vi "Instrument Manager Loop.vi"(8 "System Control":refnum<queue>, 11 "Optimizer Manager":refnum<queue>) -> (0 "error out":errorcluster)   [LabVIEW 2020, in "SQSnobFit Control Panel.lvlib" / "Instrument Manager.lvlib"]
uses:
  Instrument Manager/Instrument Manager.lvlib
  support/Message Queue/Message Cluster.ctl
  Instrument Manager/Instrument State.ctl
  <vilib>/addons/zeromq/zmq_context.lvclass
  <vilib>/addons/zeromq/zmq_socket.lvclass
  <vilib>/addons/zeromq/socket_type.ctl
  <vilib>/addons/zeromq/poll_type.ctl
  Typedefs/Best Result.ctl
  <vilib>/Utility/error.llb/Error Cluster From Error Code.vi
  <vilib>/addons/zeromq/zmq_poll_scalar.vi
  <vilib>/ErrorRing/Error Ring.xnode
  support/Message Queue/Message Queue.lvlib
  SQSnobFit Control Panel.lvlib
  <vilib>/addons/zeromq/zeromq.lvlib
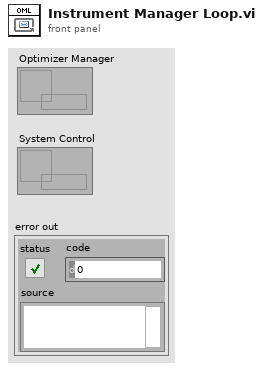
[diagram p1: front panel]
types:
  T1 = typedef "zeromq.lvlib/socket_type.ctl" = enum8{"ZMQ_PAIR", "ZMQ_PUB", "ZMQ_SUB", "ZMQ_REQ", "ZMQ_REP", "ZMQ_DEALER", "ZMQ_ROUTER", "ZMQ_PULL", "ZMQ_PUSH", "ZMQ_XPUB", "ZMQ_XSUB"}
  T2 = typedef "SQSnobFit Control Panel.lvlib/Instrument Manager.lvlib/Instrument State.ctl" = cluster{"Context":refnum<class "zmq_context.lvclass">, "Socket":refnum<class "zmq_socket.lvclass">, "Running Since":timestamp, "New Parameters (values)":cluster{"Time Stamp":timestamp, "Name":string[], "Value":dbl[]}, "Optimizer Path":path, "Running":bool, "Response Counter":u8, "Response Timeout (ms)":u32, "Response Retries":u32, "Endpoint":string, "Starting up?":bool, "New Parameters (percents)":cluster{"Time Stamp":timestamp, "Name":string[], "Value":dbl[]}, "Flow Rate Constant":dbl, "Yield":dbl, "Current Best (values)":cluster{"Parameter Names":string[], "Parameter Values":dbl[], "Function Value":dbl}}
  T3 = typedef "zeromq.lvlib/poll_type.ctl" = enum16{"None", "In", "Out", "In/Out"}
  T4 = typedef "SQSnobFit Control Panel.lvlib/Best Result.ctl" = cluster{"value":dbl, "parameters":dbl[], "history":dbl[][], "steps":dbl}
  T5 = cluster{"seconds since 1Jan1904":timestamp, string[], dbl[]}
  T6 = cluster{"Time Stamp":timestamp, "Name":string[], "Value":dbl[]}
  T7 = typedef "zeromq.lvlib/error_type.ctl" = enum16{"No Error", "EUNKNOWN", "ENOTSUP", "EPROTONOSUPPORT", "ENOBUFS", "ENETDOWN", "EADDRINUSE", "EADDRNOTAVAIL", "ECONNREFUSED", "EINPROGRESS", "ENOTSOCK", "EMSGSIZE", "EAFNOSUPPORT", "ENETUNREACH", "ECONNABORT", "ECONNRESET", "ENOTCONN", "ETIMEDOUT", "EHOSTUNREACH", "ENETRESET", "EBUSY", "EINVAL", "ENODEV", "EFAULT", "EINTR", "ENOENT", "ENOMEM", "EAGAIN", "EMFILE", "EFSM", "ENOCOMPATPROTO", "ETERM", "EMTHREAD", "Invalid"}
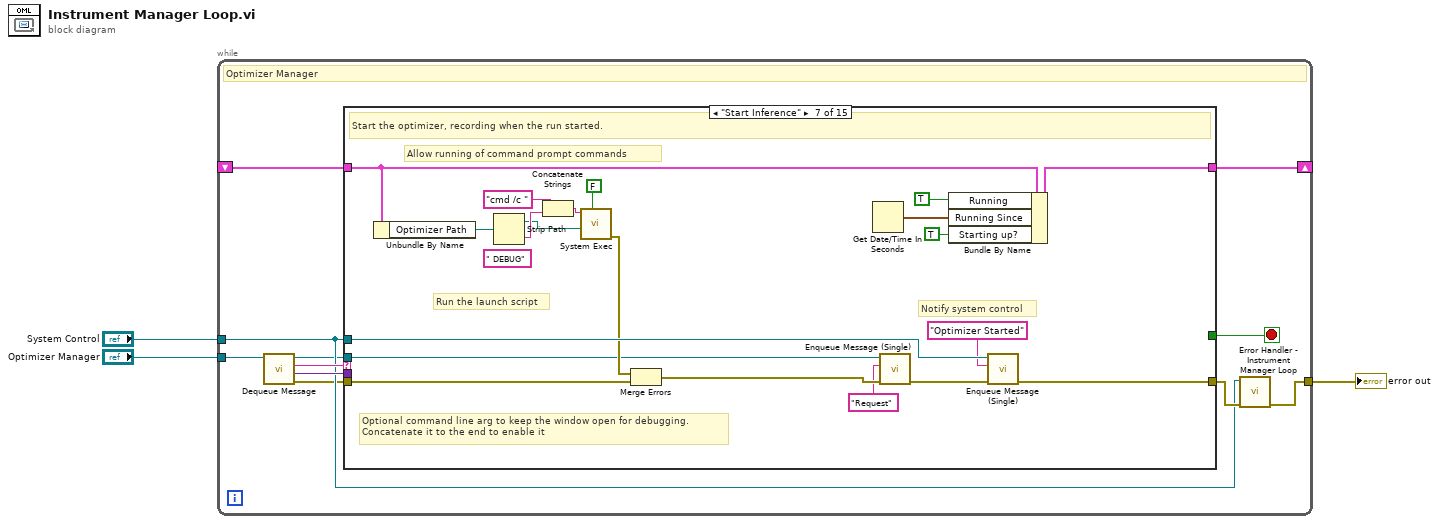
[diagram p0: block diagram]
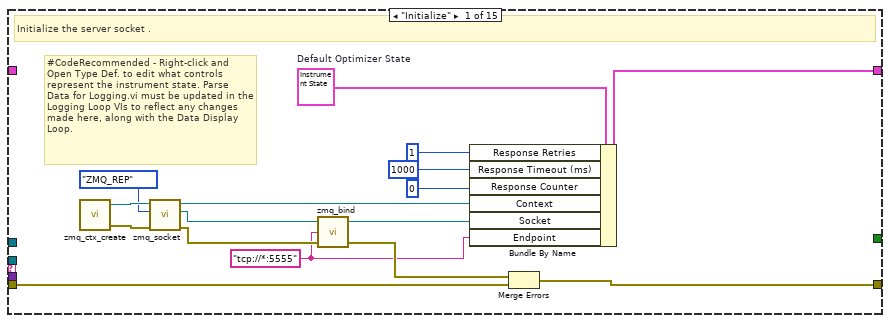
[diagram p2: hidden frame]
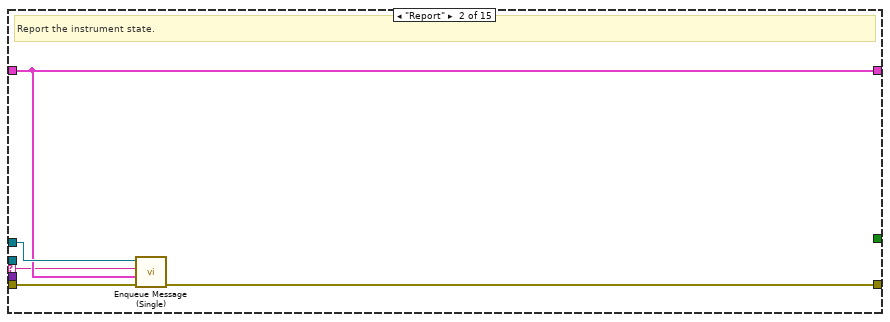
[diagram p3: hidden frame]
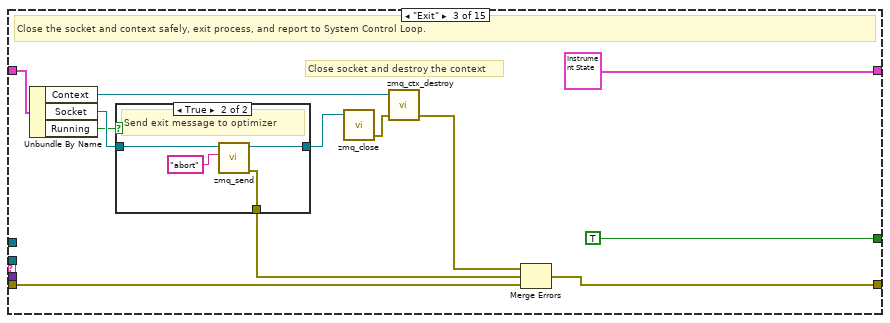
[diagram p4: hidden frame]
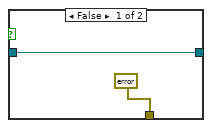
[diagram p5: hidden frame]
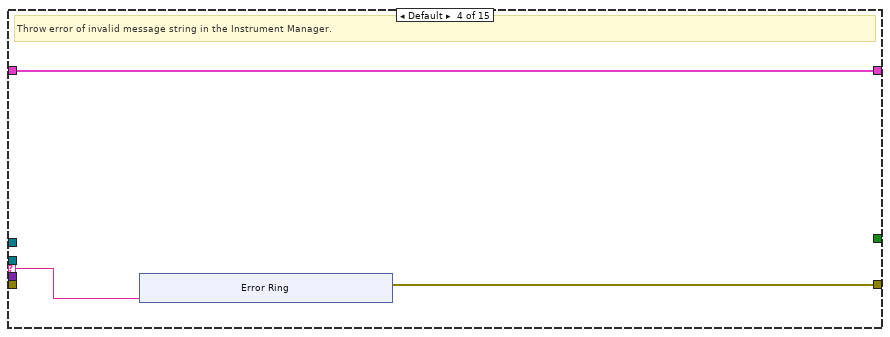
[diagram p6: hidden frame]
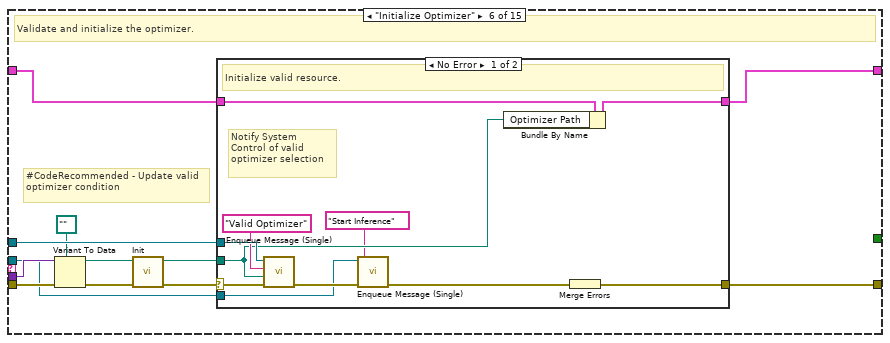
[diagram p8: hidden frame]
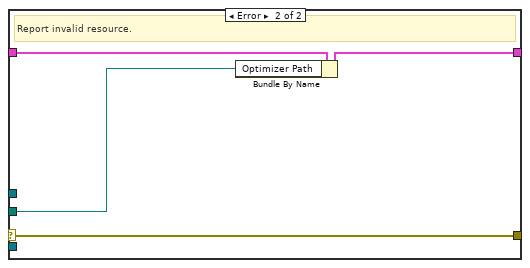
[diagram p9: hidden frame]
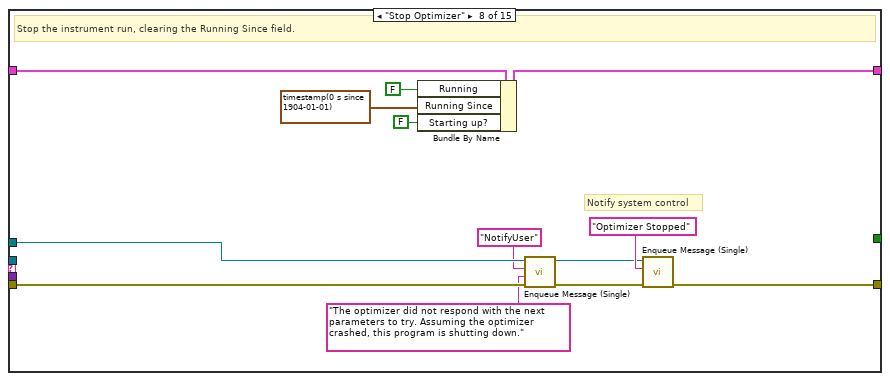
[diagram p10: hidden frame]
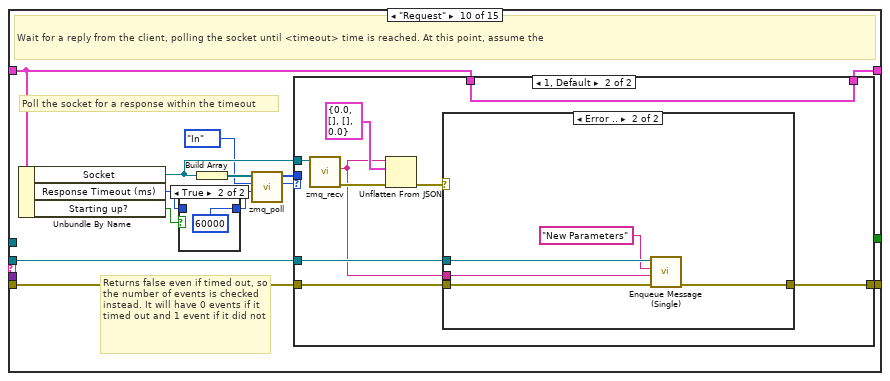
[diagram p12: hidden frame]
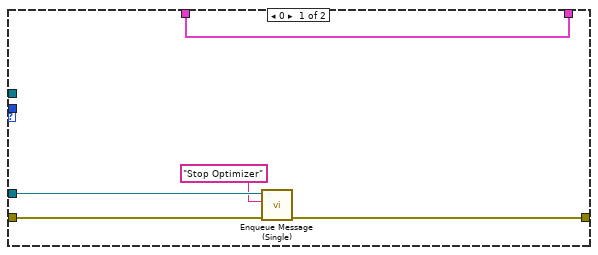
[diagram p14: hidden frame]
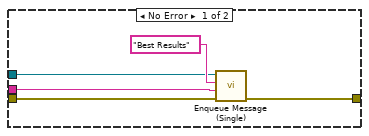
[diagram p15: hidden frame]
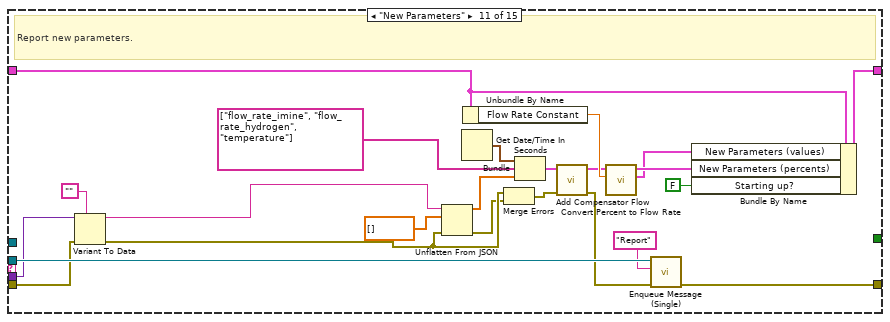
[diagram p16: hidden frame]
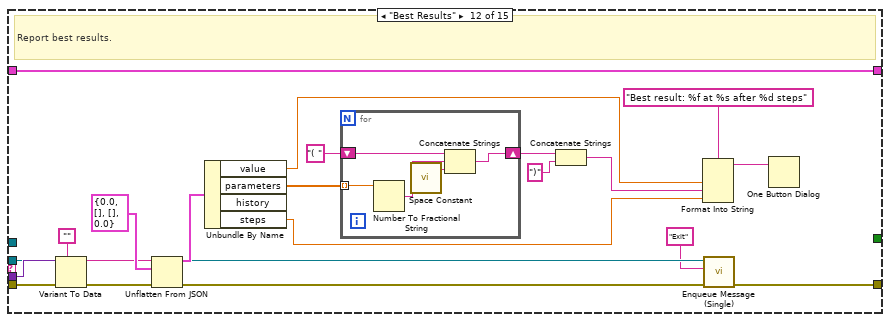
[diagram p17: hidden frame]
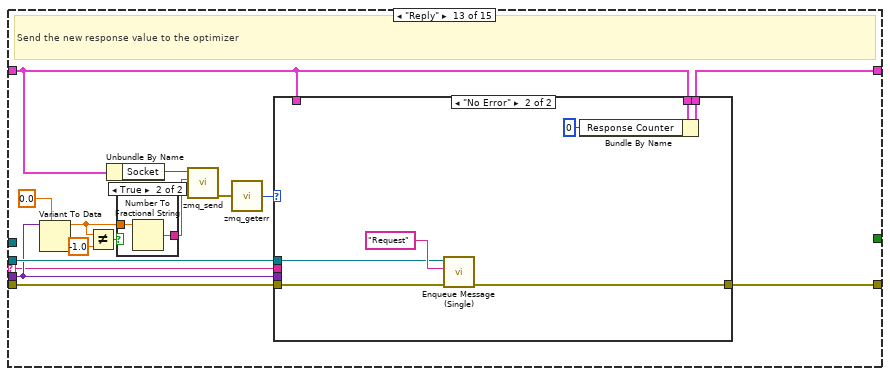
[diagram p18: hidden frame]
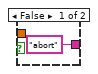
[diagram p19: hidden frame]
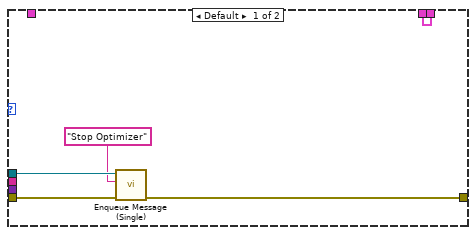
[diagram p20: hidden frame]
diagram:
  n1 = while {
    tunnel: "Optimizer Manager" -> [w14]
    tunnel: "System Control" -> [w6]
    tunnel: [w10] -> w1
    shift-right: [w8] -> _
    shift-left: _ -> [w9]
    stop <- w7 stop-if-true
    # "Optimizer Manager"
    n2 = call "Dequeue Message.vi"("Message Queue"=w14) -> ("error out"=w5:errorcluster, "Message Data"=w12:variant, "Message"=w13:string, "dup Message Queue"=w4:refnum<queue>)  [unwired: 7 in]
    n3 = case shown="\"Start Inference\"" w13 {
      selector: w13 -> [_ w31 _ w55 _ _ _ _ _ _ _ _ w220 _ _]
      tunnel: w4 -> [_ _ _ _ _ w66 w95 _ _ w134 w186 w191 w225 w258 w278]
      tunnel: w6 -> [_ w34 _ _ _ w68 w110 w117 _ _ _ _ _ w252 _]
      tunnel: w12 -> [_ _ _ _ _ w74 _ _ _ _ w173 w206 w221 w255 w285]
      tunnel: w5 -> [w30 w35 w42 _ w64 w73 w112 w118 w127 w133 w174 w209 w224 w257 w286]
      tunnel: [w24 w33 w45 w54 w64 w77 w111 w124 w127 w135 w187 w192 w219 w256 w280] -> w11
      tunnel: w9 -> [_ w32 w41 w56 w65 w76 w105 w125 w126 w139 w188 w210 w223 w246 w287]
      tunnel: [w27 w32 T2 {"Context"=refnum, "Socket"=refnum, "Running Since"=timestamp(0 s since 1904-01-01), "New Parameters (values)"={"Time Stamp"=timestamp(0 s since 1904-01-01), "Name"=[], "Value"=[]}, "Optimizer Path"=path "", "Running"=FALSE, "Response Counter"=0, "Response Timeout (ms)"=0, "Response Retries"=0, "Endpoint"="", "Starting up?"=FALSE, "New Parameters (percents)"={"Time Stamp"=timestamp(0 s since 1904-01-01), "Name"=[], "Value"=[]}, "Flow Rate Constant"=0.0, "Yield"=0.0, "Current Best (values)"={"Parameter Names"=[], "Parameter Values"=[], "Function Value"=0.0}} w56 w65 w75 w108 w122 w126 w140 w189 w210 w222 w247 w276] -> w8
      tunnel: [_ _ TRUE _ _ _ _ _ _ _ _ _ _ _ _] -> w7
      frame "Initialize" {
        w15 = "tcp://*:5555" ("endpoint")
        w28 = T2 {"Context"=refnum, "Socket"=refnum, "Running Since"=timestamp(0 s since 1904-01-01), "New Parameters (values)"={"Time Stamp"=timestamp(0 s since 1904-01-01), "Name"=[], "Value"=[]}, "Optimizer Path"=path "", "Running"=FALSE, "Response Counter"=0, "Response Timeout (ms)"=0, "Response Retries"=0, "Endpoint"="", "Starting up?"=FALSE, "New Parameters (percents)"={"Time Stamp"=timestamp(0 s since 1904-01-01), "Name"=[], "Value"=[]}, "Flow Rate Constant"=0.0, "Yield"=0.0, "Current Best (values)"={"Parameter Names"=[], "Parameter Values"=[], "Function Value"=0.0}}  # Default Optimizer State
        # "#CodeRecommended - Right-click and Open Type Def. to edit what controls represent the instrument state. Parse Data for Logging.vi must be updated in the Logging Loop VIs to reflect any changes made here, along with the Data Display Loop."
        # "Initialize the server socket ."
        n4 = call <vilib>:"zmq_ctx_create.vi"() -> ("error out"=w29:errorcluster, "context out"=w26:refnum<class "zmq_context.lvclass">)  [unwired: 4 in]
        n5 = call <vilib>:"zmq_socket.vi"("error in"=w29, "socket type"=socket_type."ZMQ_REP", "context in"=w26) -> ("error out"=w18:errorcluster, "socket out"=w17:refnum<class "zmq_socket.lvclass">, "context out"=w25:refnum<class "zmq_context.lvclass">)  [unwired: 2 in]
        n6 = call <vilib>:"zmq_bind.vi"("error in"=w18, "endpoint"=w15, "socket in"=w17) -> ("error out"=w19:errorcluster, "socket out"=w20:refnum<class "zmq_socket.lvclass">)  [unwired: 1 in]
        n7 = Bundle By Name(cluster=w28, "Response Retries"=u32 1 ("Consecutive Timeouts Before Heartbeat"), "Response Timeout (ms)"=u32 1000 ("Timeout (ms)"), "Response Counter"=u8 0 ("Consecutive Timeouts"), "Context"=w25, "Socket"=w20, "Endpoint"=w15) -> (w27:T2)
        n8 = Merge Errors(w19, w30) -> (w24:errorcluster)
      }
      frame "Report" {
        # "Report the instrument state."
        n9 = call "Enqueue Message (Single).vi"("error in (no error)"=w35, "Message Data"=w32, "Message"=w31, "Message Queue"=w34) -> ("error out"=w33:errorcluster)  [unwired: 6 in, 1 out]
      }
      frame "Exit" {
        # "Close socket and destroy the context"
        # "Close the socket and context safely, exit process, and report to System Control Loop."
        n10 = Unbundle By Name(w41) -> ("Context"=w43:refnum<class "zmq_context.lvclass">, "Socket"=w40:refnum<class "zmq_socket.lvclass">, "Running"=w36:bool)
        n11 = case shown="True" w36 {
          tunnel: w40 -> [w48 w52]
          tunnel: [w48 w51] -> w39
          tunnel: [errorcluster {"status"=FALSE, "code"=0, "source"=""} ("error out") w50] -> w37
          frame False {
          }
          frame True {
            # "Send exit message to optimizer"
            n12 = call <vilib>:"zmq_send.vi"("data"="abort", "socket in"=w52) -> ("error out"=w50:errorcluster, "socket out"=w51:refnum<class "zmq_socket.lvclass">)  [unwired: 5 in]
          }
        }
        n13 = call <vilib>:"zmq_close.vi"("socket"=w39) -> ("error out"=w44:errorcluster)  [unwired: 4 in]
        n14 = call <vilib>:"zmq_ctx_destroy.vi"("error in"=w44, "context in"=w43) -> ("error out"=w38:errorcluster)  [unwired: 3 in]
        n15 = Merge Errors(w38, w37, w42) -> (w45:errorcluster)
      }
      frame Default {
        # "Throw error of invalid message string in the Instrument Manager."
        n16 = xnode "Error Ring"("parameter 0"=w55) -> ("error out"=w54:errorcluster)
      }
      frame "--- Copy This Frame ---" {
        # "Copy this frame and add responses to instrument specific messages."
      }
      frame "Initialize Optimizer" {
        # "#CodeRecommended - Update valid optimizer condition"
        # "Validate and initialize the optimizer."
        n17 = Variant To Data(error in=w73, type=path "", Variant=w74) -> (data=w71:path, error out=w72:errorcluster)
        n18 = call "Init.vi"("error in (no error)"=w72, "optimizer path"=w71) -> ("error out"=w69:errorcluster, "optimizer path (out)"=w70:path)  [unwired: 8 in]
        n19 = case shown="No Error" w69 {
          selector: w69 -> [w87 w89]
          tunnel: w70 -> [w83 w90]
          tunnel: [w82 w89] -> w77
          tunnel: w76 -> [w88 w92]
          tunnel: [w84 w91] -> w75
          tunnel: w68 -> [w86 _]
          tunnel: w66 -> [w79 _]
          frame No Error {
            # "Notify System Control of valid optimizer selection"
            # "Initialize valid resource."
            n20 = call "Enqueue Message (Single).vi"("error in (no error)"=w87, "Message Data"=w83, "Message"="Valid Optimizer", "Message Queue"=w86) -> ("error out"=w81:errorcluster)  [unwired: 6 in, 1 out]
            n21 = call "Enqueue Message (Single).vi"("error in (no error)"=w81, "Message"="Start Inference", "Message Queue"=w79) -> ("error out"=w80:errorcluster)  [unwired: 7 in, 1 out]
            n22 = Bundle By Name(cluster=w88, "Optimizer Path"=w83) -> (w84:T2)
            n23 = Merge Errors(w80) -> (w82:errorcluster)
          }
          frame Error {
            # "Report invalid resource."
            n24 = Bundle By Name(cluster=w92, "Optimizer Path"=w90) -> (w91:T2)
          }
        }
      }
      frame "Start Inference" {
        (unwired) " DEBUG" ("string")
        # "Optional command line arg to keep the window open for debugging.\nConcatenate it to the end to enable it"
        # "Allow running of command prompt commands"
        # "Run the launch script"
        # "Notify system control"
        # "Start the optimizer, recording when the run started."
        n25 = Unbundle By Name(w105) -> ("Optimizer Path"=w102:path)
        n26 = Strip Path(path=w102) -> (stripped path=w100:path, name=w101:string)
        n27 = Concatenate Strings("cmd /c " ("string"), w101) -> (w99:string)
        n28 = call <vilib>:"System Exec.vi"("wait until completion? (T)"=FALSE, "working directory"=w100, "command line"=w99) -> ("error out"=w103:errorcluster)  [unwired: 5 in, 3 out]
        n29 = Merge Errors(w103, w112) -> (w96:errorcluster)
        n30 = Get Date/Time In Seconds() -> (seconds since 1Jan1904=w106:timestamp)
        n31 = call "Enqueue Message (Single).vi"("error in (no error)"=w96, "Message"="Request", "Message Queue"=w95) -> ("error out"=w97:errorcluster)  [unwired: 7 in, 1 out]
        n32 = Bundle By Name(cluster=w105, "Running"=TRUE, "Running Since"=w106, "Starting up?"=TRUE) -> (w108:T2)
        n33 = call "Enqueue Message (Single).vi"("error in (no error)"=w97, "Message"="Optimizer Started", "Message Queue"=w110) -> ("error out"=w111:errorcluster)  [unwired: 7 in, 1 out]
      }
      frame "Stop Optimizer" {
        # "Notify system control"
        # "Stop the instrument run, clearing the Running Since field."
        n34 = Bundle By Name(cluster=w125, "Running"=FALSE, "Running Since"=timestamp(0 s since 1904-01-01), "Starting up?"=FALSE) -> (w122:T2)
        n35 = call "Enqueue Message (Single).vi"("error in (no error)"=w118, "Message Data"="The optimizer did not respond with the next parameters to try. Assuming the optimizer crashed, this program is shutting down.", "Message"="NotifyUser", "Message Queue"=w117) -> ("error out"=w119:errorcluster, "dup Message Queue"=w116:refnum<queue>)  [unwired: 6 in]
        n36 = call "Enqueue Message (Single).vi"("error in (no error)"=w119, "Message"="Optimizer Stopped", "Message Queue"=w116) -> ("error out"=w124:errorcluster)  [unwired: 7 in, 1 out]
      }
      frame "--- Copy for Get State Messages ---" {
        # "#CodeNeeded - Use the Bundle by Name function to bundle the new state value into the Instrument State cluster."
        # "#CodeNeeded - Add instrument driver call to query the instrument state requested"
        # "Duplicate this case for messages cases that will query the instrument state."
      }
      frame "Request" {
        # "Returns false even if timed out, so the number of events is checked instead. It will have 0 events if it timed out and 1 event if it did not"
        # "Poll the socket for a response within the timeout"
        # "Wait for a reply from the client, polling the socket until <timeout> time is reached. At this point, assume the"
        n37 = Unbundle By Name(w139) -> ("Socket"=w137:refnum<class "zmq_socket.lvclass">, "Response Timeout (ms)"=w129:u32, "Starting up?"=w130:bool)
        n38 = case shown="True" w130 {
          tunnel: w129 -> [w141 _]
          tunnel: [w141 u32 60000 ("Response Timeout (ms)")] -> w128
          frame False {
          }
          frame True {
          }
        }
        n39 = Build Array(w137) -> (w138:refnum<class "zmq_socket.lvclass">[])
        n40 = call-poly <vilib>:"zmq_poll.vi"("timeout"=w128, "poll type"=poll_type."In", "sockets"=w138) -> ("nevents"=w131:i32, "polled events"=w132:T3[])  [unwired: 1 in, 2 out]
        n41 = case shown="1, Default" w131 {
          tunnel: [w147 w152] -> w140
          tunnel: w139 -> [w147 w152]
          tunnel: w137 -> [_ w156]
          tunnel: w133 -> [w146 w155]
          tunnel: [w143 w154] -> w135
          tunnel: w134 -> [w145 w153]
          tunnel: w132 -> [_ _]
          frame 0 {
            n42 = call "Enqueue Message (Single).vi"("error in (no error)"=w146, "Message"="Stop Optimizer", "Message Queue"=w145) -> ("error out"=w143:errorcluster)  [unwired: 7 in, 1 out]
          }
          frame 1, Default {
            n43 = call <vilib>:"zmq_recv.vi"("socket in"=w156) -> ("error out"=w151:errorcluster, "data"=w148:string)  [unwired: 4 in, 3 out]
            n44 = Unflatten From JSON(JSON string=w148, type and defaults=T4 {"value"=0.0, "parameters"=[], "history"=[], "steps"=0.0}, error in (no error)=w151) -> (error out=w149:errorcluster)  [unwired: 4 in, 1 out]
            n45 = case shown="Error .." w149 {
              tunnel: w155 -> [w161 w166]
              tunnel: [w160 w165] -> w154
              tunnel: w153 -> [w158 w164]
              tunnel: w148 -> [w157 w162]
              frame No Error {
                n46 = call "Enqueue Message (Single).vi"("error in (no error)"=w161, "Message Data"=w157, "Message"="Best Results", "Message Queue"=w158) -> ("error out"=w160:errorcluster)  [unwired: 6 in, 1 out]
              }
              frame Error {
                n47 = call "Enqueue Message (Single).vi"("error in (no error)"=w166, "Message Data"=w162, "Message"="New Parameters", "Message Queue"=w164) -> ("error out"=w165:errorcluster)  [unwired: 6 in, 1 out]
              }
            }
          }
        }
      }
      frame "New Parameters" {
        # "Report new parameters."
        n48 = Variant To Data(error in=w174, type="", Variant=w173) -> (data=w171:string, error out=w170:errorcluster)
        n49 = Unflatten From JSON(JSON string=w171, type and defaults=dbl[] [], error in (no error)=w170) -> (value=w180:dbl[], error out=w168:errorcluster)  [unwired: 4 in]
        n50 = Get Date/Time In Seconds() -> (seconds since 1Jan1904=w182:timestamp)
        n51 = Unbundle By Name(w188) -> ("Flow Rate Constant"=w178:dbl)
        n52 = Merge Errors(w170, w168) -> (w169:errorcluster)
        n53 = Bundle("seconds since 1Jan1904"=w182, string[] ["flow_rate_imine", "flow_rate_hydrogen", "temperature"], w180) -> (w179:T5)  [unwired: 1 in]
        n54 = call "Add Compensator Flow.vi"("error in (no error)"=w169, "New Parameters (percents)"=w179) -> ("error out"=w167:errorcluster, "New Parameters (percents) out"=w175:T6)  [unwired: 8 in]
        n55 = call "Convert Percent to Flow Rate.vi"("Flow Rate Constant"=w178, "New Parameters (percents)"=w175) -> ("New Parameters (values) out"=w176:T6, "New Parameters (percents) out"=w177:T6)  [unwired: 8 in]
        n56 = call "Enqueue Message (Single).vi"("error in (no error)"=w167, "Message"="Report", "Message Queue"=w186) -> ("error out"=w187:errorcluster)  [unwired: 7 in, 1 out]
        n57 = Bundle By Name(cluster=w188, "New Parameters (values)"=w176, "New Parameters (percents)"=w177, "Starting up?"=FALSE) -> (w189:T2)
      }
      frame "Best Results" {
        # "Report best results."
        n58 = Variant To Data(error in=w209, type="", Variant=w206) -> (data=w204:string, error out=w207:errorcluster)
        n59 = Unflatten From JSON(JSON string=w204, type and defaults=T4 {"value"=0.0, "parameters"=[], "history"=[], "steps"=0.0}, error in (no error)=w207) -> (value=w203:T4, error out=w193:errorcluster)  [unwired: 4 in]
        n60 = Unbundle By Name(w203) -> ("value"=w196:dbl, "parameters"=w201:dbl[], "steps"=w202:dbl)  [unwired: 1 out]
        n61 = for {
          tunnel: w201 -> [w213] mode=indexing
          shift-right: [w214] -> w198
          shift-left: "( " -> [w215]
          n62 = Number To Fractional String(number=w213) -> (F-format string=w212:string)  [unwired: 3 in]
          n63 = call <vilib>:"Space Constant.vi"() -> ("String"=w211:string)
          n64 = Concatenate Strings(w215, w212, w211) -> (w214:string)
        }
        n65 = Concatenate Strings(w198, ")") -> (w195:string)
        n66 = Format Into String(format string="Best result: %f at %s after %d steps", w196, w195, w202) -> (resulting string=w194:string)  [unwired: 2 in, 1 out]
        n67 = call "Enqueue Message (Single).vi"("error in (no error)"=w193, "Message"="Exit", "Message Queue"=w191) -> ("error out"=w192:errorcluster)  [unwired: 7 in, 1 out]
        n68 = One Button Dialog(message=w194) -> ()  [unwired: 1 in, 1 out]
      }
      frame "Reply" {
        # "Send the new response value to the optimizer"
        n69 = Variant To Data(type=0.0, Variant=w221) -> (data=w217:dbl)  [unwired: 1 in, 1 out]
        n70 = Not Equal?(x=w217, y=-1.0) -> (x != y?=w218:bool)
        n71 = Unbundle By Name(w223) -> ("Socket"=w230:refnum<class "zmq_socket.lvclass">)
        n72 = case shown="True" w218 {
          tunnel: w217 -> [_ w233]
          tunnel: ["abort" w232] -> w228
          frame False {
          }
          frame True {
            n73 = Number To Fractional String(number=w233) -> (F-format string=w232:string)  [unwired: 3 in]
          }
        }
        n74 = call <vilib>:"zmq_send.vi"("data"=w228, "socket in"=w230) -> ("error out"=w227:errorcluster)  [unwired: 5 in, 1 out]
        n75 = call <vilib>:"zmq_geterr.vi"("error in"=w227) -> ("type"=w226:T7)
        n76 = case shown="\"No Error\"" w226 {
          tunnel: w224 -> [w237 w243]
          tunnel: w225 -> [w238 w244]
          tunnel: w220 -> [_ _]
          tunnel: [w236 w242] -> w219
          tunnel: w223 -> [w234 w241]
          tunnel: [w234 w240] -> w222
          tunnel: w223 -> [_ _]
          tunnel: w221 -> [_ _]
          frame Default {
            n77 = call "Enqueue Message (Single).vi"("error in (no error)"=w237, "Message"="Stop Optimizer", "Message Queue"=w238) -> ("error out"=w236:errorcluster)  [unwired: 7 in, 1 out]
          }
          frame "No Error" {
            n78 = call "Enqueue Message (Single).vi"("error in (no error)"=w243, "Message"="Request", "Message Queue"=w244) -> ("error out"=w242:errorcluster)  [unwired: 7 in, 1 out]
            n79 = Bundle By Name(cluster=w241, "Response Counter"=u8 0 ("Timeout Counter")) -> (w240:T2)
          }
        }
      }
      frame "Submit Yield" {
        # "Send the new yield to the optimizer"
        n80 = Variant To Data(type=0.0, Variant=w255) -> (data=w248:dbl)  [unwired: 1 in, 1 out]
        n81 = Greater Or Equal To 0?(x=w248) -> (x >= 0?=w253:bool)
        n82 = Equal?(x=-1.0, y=w248) -> (x = y?=w250:bool)
        n83 = Or(x=w250, y=w253) -> (x .or. y?=w251:bool)
        n84 = case shown="True" w251 {
          tunnel: w258 -> [w266 _]
          tunnel: w257 -> [w265 w272]
          tunnel: [w264 w271] -> w256
          tunnel: w255 -> [w262 _]
          tunnel: w252 -> [_ w269]
          tunnel: w248 -> [w259 _]
          tunnel: w246 -> [w261 w267]
          tunnel: [w260 w267] -> w247
          frame True {
            n85 = call "Enqueue Message (Single).vi"("error in (no error)"=w265, "Message Data"=w262, "Message"="Reply", "Message Queue"=w266) -> ("error out"=w264:errorcluster)  [unwired: 6 in, 1 out]
            n86 = Bundle By Name(cluster=w261, "Yield"=w259) -> (w260:T2)
          }
          frame False {
            n87 = call "Enqueue Message (Single).vi"("error in (no error)"=w272, "Message Data"="Invalid yield. Please use a positive number.", "Message"="NotifyUser", "Message Queue"=w269) -> ("error out"=w271:errorcluster)  [unwired: 6 in, 1 out]
          }
        }
      }
      frame "Flow Rate Changed" {
        # "Change the constant flow rate"
        n88 = Variant To Data(error in=w286, type=0.0, Variant=w285) -> (data=w283:dbl, error out=w281:errorcluster)
        n89 = Bundle By Name(cluster=w287, "Flow Rate Constant"=w283) -> (w275:T2)
        n90 = Unbundle By Name(w275) -> ("New Parameters (percents)"=w274:T6, "Flow Rate Constant"=w277:dbl)
        n91 = call "Convert Percent to Flow Rate.vi"("Flow Rate Constant"=w277, "New Parameters (percents)"=w274) -> ("New Parameters (values) out"=w273:T6, "New Parameters (percents) out"=w282:T6)  [unwired: 8 in]
        n92 = Bundle By Name(cluster=w275, "New Parameters (percents)"=w282, "New Parameters (values)"=w273) -> (w276:T2)
        n93 = call "Enqueue Message (Single).vi"("error in (no error)"=w281, "Message"="Report", "Message Queue"=w278) -> ("error out"=w280:errorcluster)  [unwired: 7 in, 1 out]
      }
    }
    n94 = call "Error Handler - Instrument Manager Loop.vi"("error in (no error)"=w11, "Message Queue"=w6) -> ("dup error in"=w10:errorcluster)  [unwired: 8 in, 1 out]
  }
  "error out" <- w1
